vi "SLSC Create Status.vi"() -> (3 "Outgoing configuration":T3(array[cluster])=[{"Channel Name"="LED1_Green", "SLSC Name"="Bool.LED1.NI.GreenBool", "Channel"={"Type"=enum."Input", "Units"="", "Default Value"=1.0, "Faultable"=FALSE, "Scalable"=FALSE}}, {"Channel Name"="Scratchpad8", "SLSC Name"="U32.Scratchpad8.NI.Scratchpad.AsUInt32.U8", "Channel"={"Type"=enum."Input", "Units"="", "Default Value"=12.0, "Faultable"=FALSE, "Scalable"=FALSE}}])   [LabVIEW 2015, in "SLSC CD System Explorer.lvlib"]
uses:
  SLSC CD System Explorer.lvlib
  <vilib>/NI Veristand/Custom Device API/Custom Device Channel.ctl
  <vilib>/NI Veristand/Custom Device API/Custom Device Channel Type.ctl
  <vilib>/NI VeriStand/Custom Device API/Custom Device API.lvlib
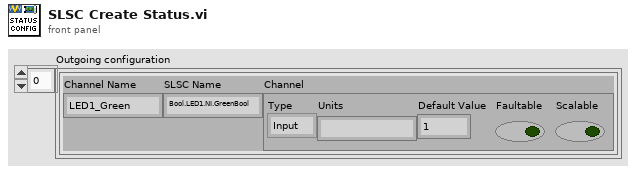
[diagram p1: front panel]
types:
  T1 = typedef "Custom Device API.lvlib/Custom Device Channel.ctl" = cluster{"Type":T2, "Units":string, "Default Value":dbl, "Faultable":bool, "Scalable":bool}
  T2 = typedef "Custom Device API.lvlib/Custom Device Channel Type.ctl" = enum16{"Input", "Output"}
  T3 = cluster{"Channel Name":string, "SLSC Name":string, "Channel":T1}[]
  T4 = cluster{"Channel Name":string, "SLSC Name":string, "Configuration":T1}[]
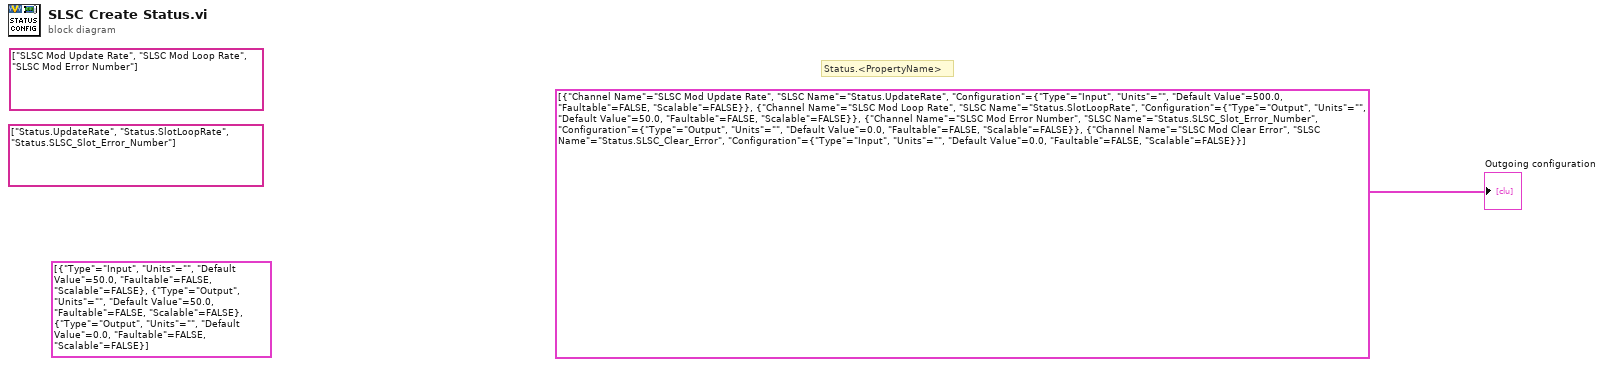
[diagram p0: block diagram]
diagram:
  (unwired) T1[] [{"Type"=enum."Input", "Units"="", "Default Value"=50.0, "Faultable"=FALSE, "Scalable"=FALSE}, {"Type"=enum."Output", "Units"="", "Default Value"=50.0, "Faultable"=FALSE, "Scalable"=FALSE}, {"Type"=enum."Output", "Units"="", "Default Value"=0.0, "Faultable"=FALSE, "Scalable"=FALSE}]
  (unwired) string[] ["SLSC Mod Update Rate", "SLSC Mod Loop Rate", "SLSC Mod Error Number"]
  (unwired) string[] ["Status.UpdateRate", "Status.SlotLoopRate", "Status.SLSC_Slot_Error_Number"]
  # "Status.<PropertyName>"
  "Outgoing configuration" <- T4 [{"Channel Name"="SLSC Mod Update Rate", "SLSC Name"="Status.UpdateRate", "Configuration"={"Type"=enum."Input", "Units"="", "Default Value"=500.0, "Faultable"=FALSE, "Scalable"=FALSE}}, {"Channel Name"="SLSC Mod Loop Rate", "SLSC Name"="Status.SlotLoopRate", "Configuration"={"Type"=enum."Output", "Units"="", "Default Value"=50.0, "Faultable"=FALSE, "Scalable"=FALSE}}, {"Channel Name"="SLSC Mod Error Number", "SLSC Name"="Status.SLSC_Slot_Error_Number", "Configuration"={"Type"=enum."Output", "Units"="", "Default Value"=0.0, "Faultable"=FALSE, "Scalable"=FALSE}}, {"Channel Name"="SLSC Mod Clear Error", "SLSC Name"="Status.SLSC_Clear_Error", "Configuration"={"Type"=enum."Input", "Units"="", "Default Value"=0.0, "Faultable"=FALSE, "Scalable"=FALSE}}]
